vi "Reset.vi"(8 "error in (no error)":errorcluster, 11 "ChromaAcLoad in":refnum<class "ChromaAcLoad.lvclass">) -> (0 "error out":errorcluster, 3 "ChromaAcLoad out":refnum<class "ChromaAcLoad.lvclass">)   [LabVIEW 2018, in "AcPwrPlugins.lvlib" / "ChromaAcLoad.lvclass"]
doc: "This VI resets the instrument to a known state and sends initialization commands to the instrument."
uses:
  ChromaAcLoad.lvclass
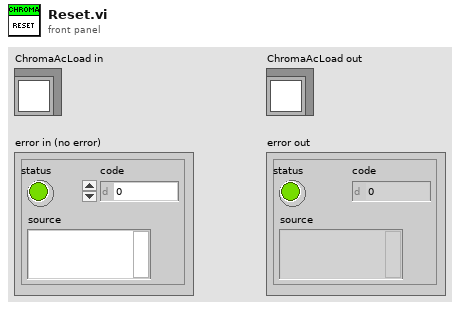
[diagram p1: front panel]
types:
  T1 = typedef "AcPwrPlugins.lvlib/ChromaAcLoad.lvclass/Device(s)Settings.ctl" = cluster{"Configuration Mode":T2, "Phases":cluster{"Handle":string, "Name":string, "Phase Select":i32, "Instrument Options":string, "id query (T)":bool, "reset device (T)":bool, "Load Short Circuited":bool, "Line Synchronization":bool, "Load Current (A/Arms)":dbl, "Load Voltage (V/Vrms)":dbl, "Load Power (W)":dbl, "Load Resistance (Ohms)":dbl, "Load Current Peak Limit (A)":dbl, "Load Current Limit (A/Arms)":dbl, "Load Power Limit (W)":dbl, "Synch Frequency (Hz)":dbl, "Priority":enum16{"CF Only", "PF Only", "Both (CF)", "Both (PF)"}, "Crest Factor":dbl, "Power Factor":dbl, "Slew Rate":cluster{"Rise Slew Rate (A/ms)":i32, "Fall Slew Rate (A/ms)":i32}, "LC/RLC Mode":cluster{"Capacitance (uF)":i32, "Inductance (uH)":i32, "Series Resistance (Ohm)":dbl, "Parallel Resistance (Ohm)":dbl}, "Timing":cluster{"TimingOn":enum16{""}, "Hours":u32, "Minutes":u32, "Seconds":dbl, "CutoffVoltage":dbl}, "Connected":bool}[], "MeasName":string}
  T2 = typedef "ConfigMode.ctl" = enum16{"Constant Voltage (DC)", "Constant Power (DC)", "Constant Power (AC)", "Constant Current (DC)", "Constant Current (AC)", "Constant Resistance (DC)", "Constant Resistance (AC)", "Rectified Mode (DC)", "Inrush (AC)", "RLC CP (AC)", "RLC (AC)"}
  T3 = typedef "AcPwrPlugins.lvlib/ChromaAcLoad.lvclass/Measurements.ctl" = cluster{"Handle":string, "Name":string, "Enabled":bool, "Measurement Value":dbl, "Hold Peak Current Measurement":bool, "btnMeasFetch":bool, "ProtectionStatusString":string, "Measurement Type":T4}[]
  T4 = typedef "AcPwrPlugins.lvlib/ChromaAcLoad.lvclass/MeasurementType.ctl" = enum16{"Voltage (Vrms or V)", "Current (Arms or A)", "Power (W)", "Peak Voltage (V)", "Peak Current (A)", "Peak Power (W)", "Frequency (Hz)", "Resistance (Ohms)", "Voltage Overshoot (V)", "Positive Peak Current (A)", "Voltage Undershoot (V)", "Negative Peak Current (A)", "Apparent Power (VA)", "Reacitive Power (VAR)", "Voltage THD", "Power Factor", "Current's Crest Factor"}
  T5 = cluster{"Handle":string, "Name":string, "Phase Select":i32, "Instrument Options":string, "id query (T)":bool, "reset device (T)":bool, "Load Short Circuited":bool, "Line Synchronization":bool, "Load Current (A/Arms)":dbl, "Load Voltage (V/Vrms)":dbl, "Load Power (W)":dbl, "Load Resistance (Ohms)":dbl, "Load Current Peak Limit (A)":dbl, "Load Current Limit (A/Arms)":dbl, "Load Power Limit (W)":dbl, "Synch Frequency (Hz)":dbl, "Priority":enum16{"CF Only", "PF Only", "Both (CF)", "Both (PF)"}, "Crest Factor":dbl, "Power Factor":dbl, "Slew Rate":cluster{"Rise Slew Rate (A/ms)":i32, "Fall Slew Rate (A/ms)":i32}, "LC/RLC Mode":cluster{"Capacitance (uF)":i32, "Inductance (uH)":i32, "Series Resistance (Ohm)":dbl, "Parallel Resistance (Ohm)":dbl}, "Timing":cluster{"TimingOn":enum16{""}, "Hours":u32, "Minutes":u32, "Seconds":dbl, "CutoffVoltage":dbl}, "Connected":bool}[]
  T6 = cluster{"Handle":string, "Name":string, "Phase Select":i32, "Instrument Options":string, "id query (T)":bool, "reset device (T)":bool, "Load Short Circuited":bool, "Line Synchronization":bool, "Load Current (A/Arms)":dbl, "Load Voltage (V/Vrms)":dbl, "Load Power (W)":dbl, "Load Resistance (Ohms)":dbl, "Load Current Peak Limit (A)":dbl, "Load Current Limit (A/Arms)":dbl, "Load Power Limit (W)":dbl, "Synch Frequency (Hz)":dbl, "Priority":enum16{"CF Only", "PF Only", "Both (CF)", "Both (PF)"}, "Crest Factor":dbl, "Power Factor":dbl, "Slew Rate":cluster{"Rise Slew Rate (A/ms)":i32, "Fall Slew Rate (A/ms)":i32}, "LC/RLC Mode":cluster{"Capacitance (uF)":i32, "Inductance (uH)":i32, "Series Resistance (Ohm)":dbl, "Parallel Resistance (Ohm)":dbl}, "Timing":cluster{"TimingOn":enum16{""}, "Hours":u32, "Minutes":u32, "Seconds":dbl, "CutoffVoltage":dbl}, "Connected":bool}
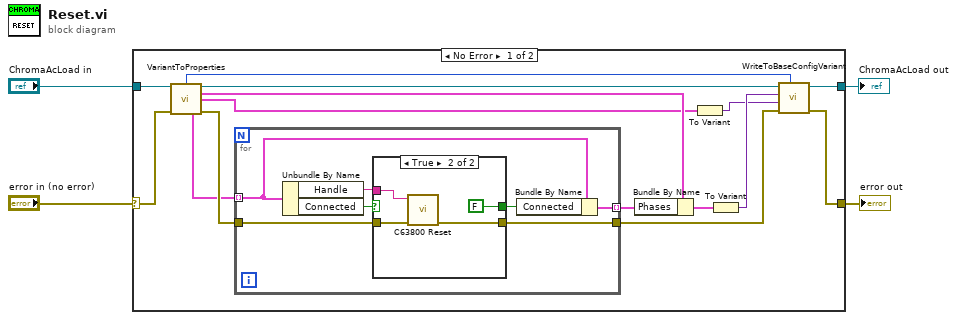
[diagram p0: block diagram]
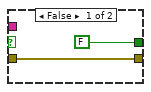
[diagram p2: hidden frame]
diagram:
  n1 = case shown="No Error" "error in (no error)" {
    selector: "error in (no error)" -> [w17 w33]
    tunnel: "ChromaAcLoad in" -> [w16 w34]
    tunnel: [w13 w34] -> w2
    tunnel: [w12 w33] -> w1
    frame No Error {
      n2 = call "VariantToProperties.vi"("ChromaAcLoad"=w16, "error in (no error)"=w17) -> ("ChromaAcLoad"=w14:refnum<class "ChromaAcLoad.lvclass">, "Device Properties"=w9:T1, "Meas"=w7:T3, "Measurement Refresh Time (ms)"=w5:u32, "Phases"=w8:T5, "error out"=w15:errorcluster)  [unwired: 7 in, 1 out]
      n3 = for {
        tunnel: w8 -> [w24] mode=indexing
        tunnel: w15 -> [w26]
        tunnel: [w20] -> w18 mode=indexing
        tunnel: [w25] -> w11
        n4 = Unbundle By Name(w24) -> ("Handle"=w21:string, "Connected"=w22:bool)
        n5 = case shown="True" w22 {
          tunnel: w26 -> [w28 w29]
          tunnel: [w28 w30] -> w25
          tunnel: w21 -> [_ w31]
          tunnel: [FALSE FALSE] -> w23
          frame False {
          }
          frame True {
            n6 = call <instrlib>:"C63800 Reset.vi"("error in (no error)"=w29, "Instrument Handle"=w31) -> ("error out"=w30:errorcluster)  [unwired: 8 in, 1 out]
          }
        }
        n7 = Bundle By Name(cluster=w24, "Connected"=w23) -> (w20:T6)
      }
      n8 = Bundle By Name(cluster=w9, "Phases"=w18) -> (w19:T1)
      n9 = To Variant(anything=w7) -> (Variant=w6:variant)
      n10 = To Variant(anything=w19) -> (Variant=w10:variant)
      n11 = call-dynamic "WriteToBaseConfigVariant.vi"("Measurement Refresh Time (ms)"=w5, "error in (no error)"=w11, "Meas"=w6, "Config"=w10, "ChromaAcLoad in"=w14) -> ("error out"=w12:errorcluster, "ChromaAcLoad out"=w13:refnum<class "ChromaAcLoad.lvclass">)  [unwired: 5 in]
    }
    frame Error {
    }
  }
  "error out" <- w1
  "ChromaAcLoad out" <- w2
